vi "Read.vi"(11 "Logs List Value in":refnum<class "Logs List Value.lvclass">) -> (2 "Logs":string[](array[string]))   [LabVIEW 2020, in "VolatusData.lvlib" / "Logs List Value.lvclass"]
uses:
  Logs List Value.lvclass
  Logs List Value.lvclass/Logs List Value.ctl
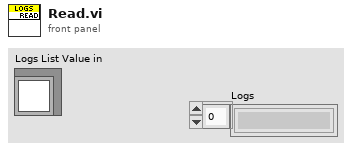
[diagram p1: front panel]
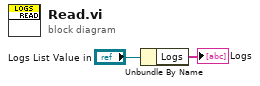
[diagram p0: block diagram]
diagram:
  n1 = Unbundle By Name("Logs List Value in") -> ("Logs"=→"Logs":string[])
